vi "libssh2_sftp_rename.vi"(8 "error in (no error)":errorcluster, 9 "destination file":string, 10 "source file":string, 11 "sftp":T1) -> (0 "error out":errorcluster)   [LabVIEW 2013, in "libssh2.lvlib"]
doc: "Rename a file or directory."
uses:
  libssh2.lvlib
  SFTP Refnum.ctl
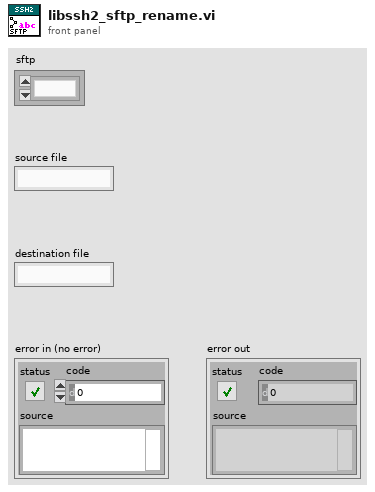
[diagram p1: front panel]
types:
  T1 = typedef "libssh2.lvlib/SFTP Refnum.ctl" = refnum<k1>
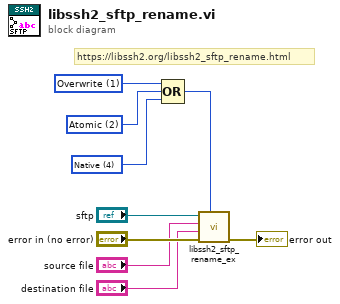
[diagram p0: block diagram]
diagram:
  w2 = 4 items=["Overwrite"=1, "Atomic"=2, "Native"=4] ("flags")
  w3 = 2 items=["Overwrite"=1, "Atomic"=2, "Native"=4] ("flags")
  w4 = 1 items=["Overwrite"=1, "Atomic"=2, "Native"=4] ("flags")
  # "https://libssh2.org/libssh2_sftp_rename.html"
  n1 = Compound Arithmetic op=OR(w4, w3, w2) -> (w1:i32)
  n2 = call "libssh2_sftp_rename_ex.vi"("flags"=w1, "error in (no error)"="error in (no error)", "destination file"="destination file", "source file"="source file", "sftp"="sftp") -> ("error out"=→"error out":errorcluster)  [unwired: 6 in]
